vi "getState.vi"(8 "error in (no error)":errorcluster, 11 "ConfiguringState in":refnum<class "ConfiguringState.lvclass">) -> (0 "error out":errorcluster, 2 "State":T1, 3 "ConfiguringState out":refnum<class "ConfiguringState.lvclass">)   [LabVIEW 2016, in "ConfiguringState.lvclass"]
uses:
  ConfiguringState.lvclass
  internalState.ctl
  Electrometer.lvclass
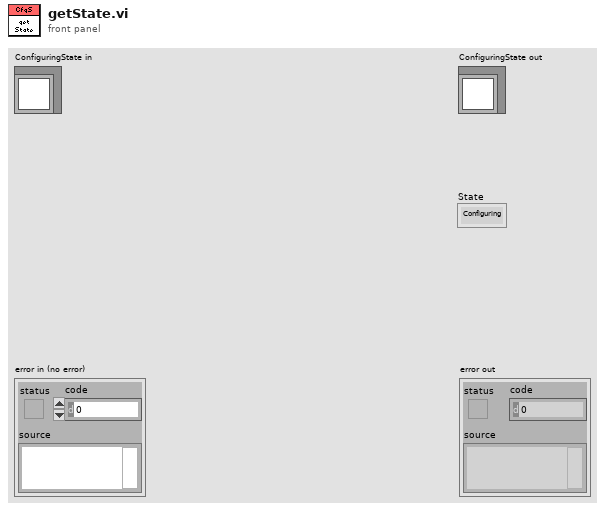
[diagram p1: front panel]
types:
  T1 = typedef "Electrometer.lvclass/internalState.ctl" = enum16{"Configuring", "Ready", "Reading"}
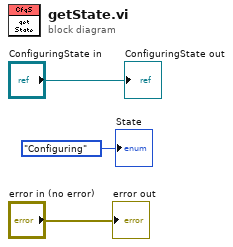
[diagram p0: block diagram]
diagram:
  "error out" <- "error in (no error)"
  "ConfiguringState out" <- "ConfiguringState in"
  "State" <- internalState."Configuring" ("State")
